vi "基础 3.vi"() -> ()   [LabVIEW 2014]
panel:
  out "x>y?":bool
  in  "y":dbl
  in  "x":dbl
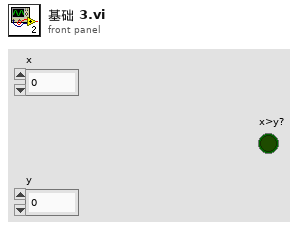
[diagram p1: front panel]
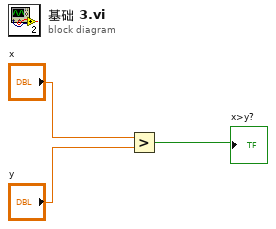
[diagram p0: block diagram]
diagram:
  n1 = Greater?(x="x", y="y") -> (0:→"x>y?":bool)
